vi "Update TaskView.vi"(8 "error in (no error)":errorcluster, 11 "BuildServer in":refnum<class "BuildServer.lvclass">) -> (0 "error out":errorcluster, 3 "BuildServer out":refnum<class "BuildServer.lvclass">)   [LabVIEW 2017, in "BuildServer.lvlib" / "BuildServer.lvclass"]
uses:
  BuildServer.lvclass
  <vilib>/Ekim/LUT/LUT/LUT.lvclass
  Classes/Task Interface/Task/Task.lvclass
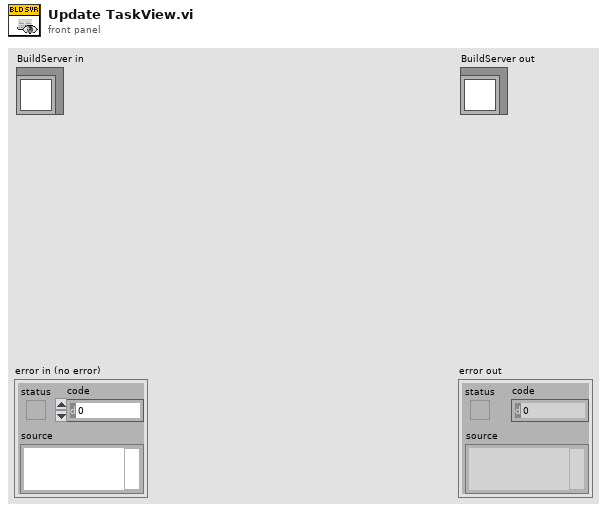
[diagram p1: front panel]
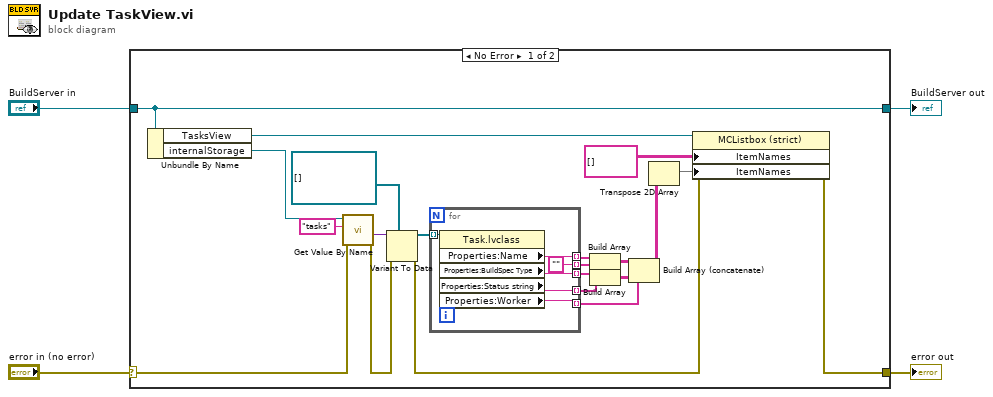
[diagram p0: block diagram]
diagram:
  n1 = case shown="No Error" "error in (no error)" {
    selector: "error in (no error)" -> [w9 w33]
    tunnel: [w7 w33] -> w3
    tunnel: [w16 w32] -> w1
    tunnel: "BuildServer in" -> [w16 w32]
    frame No Error {
      n2 = Unbundle By Name(w16) -> ("TasksView"=w17:refnum<vi>, "internalStorage"=w11:refnum<class "LUT.lvclass">)
      n3 = call <vilib>:"Get Value By Name.vi"("error in (no error)"=w9, "Name"="tasks", "LUT in"=w11) -> ("error out"=w10:errorcluster, "Value"=w14:variant)  [unwired: 5 in, 2 out]
      n4 = Variant To Data(error in=w10, type=refnum<class "Task.lvclass">[] [] ("Selected Tasks"), Variant=w14) -> (data=w12:refnum<class "Task.lvclass">[], error out=w8:errorcluster)
      n5 = for {
        tunnel: w12 -> [w31] mode=indexing
        tunnel: [w30] -> w25 mode=indexing
        tunnel: [w29] -> w23 mode=indexing
        tunnel: [w28] -> w22 mode=indexing
        tunnel: [""] -> w24 mode=indexing
        tunnel: [w26] -> w5 mode=indexing
        n6 = property class="Task.lvclass"(reference=w31) -> ("Properties:Name"=w30:string, "Properties:BuildSpec Type"=w29:string, "Properties:Status string"=w28:string, "Properties:Worker"=w26:string)  [unwired: 1 in, 2 out]
      }
      n7 = Build Array(w25, w24) -> (w21:string[][])
      n8 = Build Array(w23, w22) -> (w20:string[][])
      n9 = Build Array (concatenate)(w21, w20, w5) -> (w19:string[][])
      n10 = Transpose 2D Array(2D array=w19) -> (transposed array=w18:string[][])
      n11 = property class="MCListbox (strict)"(reference=w17, error in=w8, "ItemNames"=string[][] [] ("Item Names"), "ItemNames"=w18) -> (error out=w7:errorcluster)  [unwired: 1 out]
    }
    frame Error {
    }
  }
  "error out" <- w3
  "BuildServer out" <- w1
